vi "TCP Daemon.vi"(8 "UUID":string, 9 "Data Model":refnum<class "Device Data Model.lvclass">, 10 "transmission data unit":refnum<class "Transmission Data Unit.lvclass">, 11 "TCP slave in":refnum<class "TCP Slave.lvclass">) -> ()   [LabVIEW 2021, in "TCP Slave.lvclass"]
doc: "This daemon waits for new connections and launches connection handlers as needed. It also obtains a local reference to the quit notification, and waits for that to occur."
uses:
  TCP Slave.lvclass
  TCP Slave.lvclass/TCP Slave.ctl
  daemon status.ctl
  Network Slave.lvclass
  Listener State.ctl
  D:/my_projects/projects/Algorithms/Labview/21/Modbus_v21/Network Protocol/Network Slave/Network Slave.lvclass
  D:/my_projects/projects/Algorithms/Labview/21/Modbus_v21/Network Protocol/Network Protocol.lvclass
  D:/my_projects/projects/Algorithms/Labview/21/Modbus_v21/Network Protocol/Network Slave/TCP/TCP Slave.lvclass
  Data Model/Device Data Model.lvclass
  Transmission Data Unit/Transmission Data Unit.lvclass
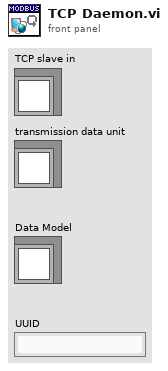
[diagram p1: front panel]
types:
  T1 = typedef "TCP Slave.lvclass/Listener State.ctl" = enum16{"Check Notifier", "Check for Available Connection Slot", "Wait on Connection", "Quit"}
  T2 = typedef "Network Slave.lvclass/daemon status.ctl" = enum16{"Not Started", "Running", "Error", "Stopped"}
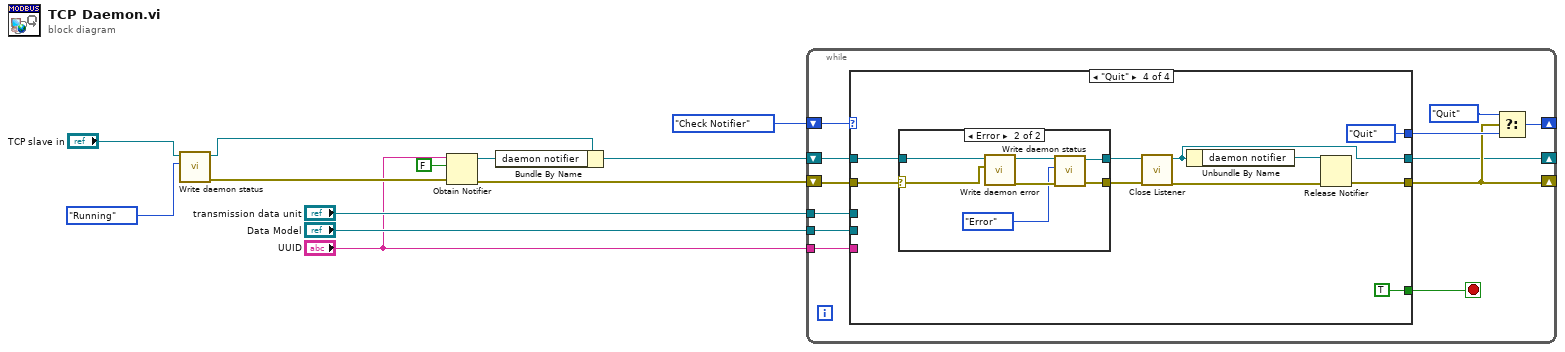
[diagram p0: block diagram]
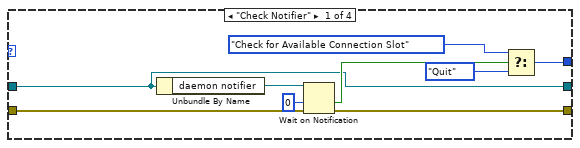
[diagram p2: hidden frame]
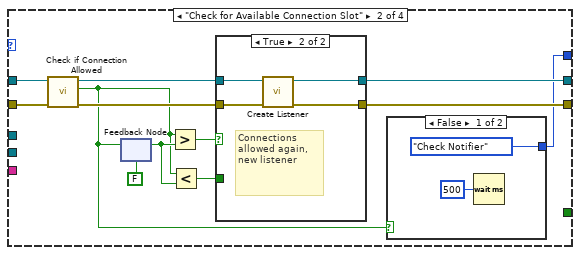
[diagram p3: hidden frame]
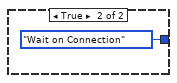
[diagram p4: hidden frame]
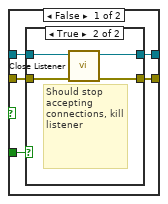
[diagram p5: hidden frame]
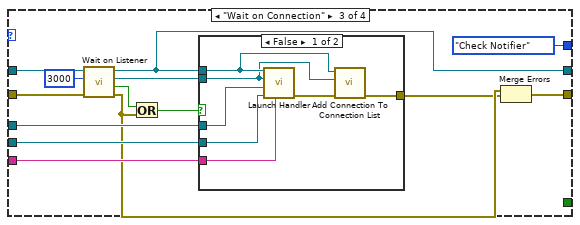
[diagram p7: hidden frame]
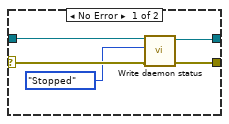
[diagram p9: hidden frame]
diagram:
  n1 = call "Write daemon status.vi"("daemon status"=daemon_status."Running", "Network Slave in"="TCP slave in") -> ("error out"=w6:errorcluster, "Network Slave out"=w7:refnum<class "TCP Slave.lvclass">)  [unwired: 8 in]
  n2 = Obtain Notifier(name (unnamed)="UUID", notification data type=FALSE, error in (no error)=w6) -> (notifier out=w10:refnum<notifier>, error out=w8:errorcluster)  [unwired: 1 in, 1 out]
  n3 = Bundle By Name(cluster=w7, "daemon notifier"=w10) -> (w9:refnum<class "TCP Slave.lvclass">)
  n4 = while {
    shift-right: [w22] -> _
    shift-left: Listener_State."Check Notifier" -> [w24]
    tunnel: "UUID" -> [w19]
    tunnel: "Data Model" -> [w18]
    tunnel: "transmission data unit" -> [w17]
    shift-right: [w16] -> _
    shift-left: w8 -> [w15]
    shift-right: [w13] -> _
    shift-left: w9 -> [w23]
    stop <- w14 stop-if-true
    n5 = case shown="\"Quit\"" w24 {
      tunnel: w23 -> [w25 w44 w76 w93]
      tunnel: [w32 w38 w66 w90] -> w16
      tunnel: [w27 w34 Listener_State."Check Notifier" Listener_State."Quit"] -> w20
      tunnel: w19 -> [_ _ w71 _]
      tunnel: w18 -> [_ _ w70 _]
      tunnel: w17 -> [_ _ w69 _]
      tunnel: w15 -> [w26 w45 w68 w94]
      tunnel: [_ _ _ TRUE] -> w14
      tunnel: [w25 w39 w67 w85] -> w13
      frame "Check Notifier" {
        n6 = Unbundle By Name(w25) -> ("daemon notifier"=w33:refnum<notifier>)
        n7 = Wait on Notification(notifier=w33, timeout in ms (-1)=0, error in (no error)=w26) -> (timed out?=w31:bool, error out=w32:errorcluster)  [unwired: 1 in, 2 out]
        n8 = Select(t=Listener_State."Check for Available Connection Slot", s=w31, f=Listener_State."Quit") -> (s? t:f=w27:T1)
      }
      frame "Check for Available Connection Slot" {
        n9 = call "Check if Connection Allowed.vi"("error in (no error)"=w45, "TCP Slave in"=w44) -> ("error out"=w41:errorcluster, "Connection Allowed"=w35:bool, "TCP Slave out"=w40:refnum<class "TCP Slave.lvclass">)  [unwired: 7 in]
        n10 = feedback-in #1(w35) -> ()
        n11 = feedback #1(FALSE) -> (w37:bool)
        n12 = Greater?(x=w35, y=w37) -> (0:w42:bool)
        n13 = Less?(x=w35, y=w37) -> (x < y?=w36:bool)
        n14 = case shown="True" w42 {
          tunnel: w41 -> [w51 w62]
          tunnel: w40 -> [w52 w63]
          tunnel: [w49 w61] -> w39
          tunnel: [w50 w60] -> w38
          tunnel: w36 -> [w53 _]
          frame False {
            n15 = case shown="True" w53 {
              tunnel: w52 -> [w55 w59]
              tunnel: w51 -> [w54 w58]
              tunnel: [w54 w57] -> w50
              tunnel: [w55 w56] -> w49
              frame False {
              }
              frame True {
                # "Should stop accepting connections, kill listener"
                n16 = call "Close Listener.vi"("error in"=w58, "TCP slave in"=w59) -> ("error out"=w57:errorcluster, "TCP slave out"=w56:refnum<class "TCP Slave.lvclass">)  [unwired: 8 in]
              }
            }
          }
          frame True {
            # "Connections allowed again, new listener"
            n17 = call "Create Listener.vi"("error in"=w62, "TCP slave in"=w63) -> ("error out"=w60:errorcluster, "TCP slave out"=w61:refnum<class "TCP Slave.lvclass">)  [unwired: 8 in]
          }
        }
        n18 = case shown="False" w35 {
          tunnel: [Listener_State."Check Notifier" Listener_State."Wait on Connection"] -> w34
          frame False {
            n19 = Wait (ms)(milliseconds to wait=u32 500) -> ()  [unwired: 1 out]
          }
          frame True {
          }
        }
      }
      frame "Wait on Connection" {
        n20 = call-dynamic "Wait on Listener.vi"("error in"=w68, "timeout ms (wait forever: -1)"=3000, "TCP slave in"=w76) -> ("error out"=w65:errorcluster, "Timed Out"=w74:bool, "connection reference"=w72:refnum<data-value>, "TCP slave out"=w67:refnum<class "TCP Slave.lvclass">)  [unwired: 5 in]
        n21 = Or(x=w74, y=w65) -> (x .or. y?=w73:bool)
        n22 = case shown="False" w73 {
          tunnel: w72 -> [w78 _]
          tunnel: w67 -> [w79 _]
          tunnel: w71 -> [w84 _]
          tunnel: w70 -> [w83 _]
          tunnel: w69 -> [w82 _]
          tunnel: [w81 _] -> w64
          frame False {
            n23 = call "Launch Handler.vi"("UUID"=w84, "Data Model"=w83, "transmission data unit"=w82, "connection reference"=w78, "TCP slave"=w79) -> ("error out"=w80:errorcluster)  [unwired: 6 in]
            n24 = call "Add Connection To Connection List.vi"("error in"=w80, "data value reference"=w78, "TCP Slave in"=w79) -> ("error out"=w81:errorcluster)  [unwired: 8 in]
          }
          frame True {
          }
        }
        n25 = Merge Errors(w65, w64) -> (w66:errorcluster)
      }
      frame "Quit" {
        n26 = case shown="Error" w94 {
          selector: w94 -> [w96 w101]
          tunnel: [w97 w103] -> w92
          tunnel: w93 -> [w99 w106]
          tunnel: [w98 w104] -> w91
          frame No Error {
            n27 = call "Write daemon status.vi"("error in (no error)"=w96, "daemon status"=daemon_status."Stopped", "Network Slave in"=w99) -> ("error out"=w97:errorcluster, "Network Slave out"=w98:refnum<class "TCP Slave.lvclass">)  [unwired: 7 in]
          }
          frame Error {
            n28 = call "Write daemon error.vi"("daemon error"=w101, "Network Slave in"=w106) -> ("error out"=w102:errorcluster, "Network Slave out"=w105:refnum<class "TCP Slave.lvclass">)  [unwired: 8 in]
            n29 = call "Write daemon status.vi"("error in (no error)"=w102, "daemon status"=daemon_status."Error", "Network Slave in"=w105) -> ("error out"=w103:errorcluster, "Network Slave out"=w104:refnum<class "TCP Slave.lvclass">)  [unwired: 7 in]
          }
        }
        n30 = call "Close Listener.vi"("error in"=w92, "TCP slave in"=w91) -> ("error out"=w86:errorcluster, "TCP slave out"=w85:refnum<class "TCP Slave.lvclass">)  [unwired: 8 in]
        n31 = Unbundle By Name(w85) -> ("daemon notifier"=w87:refnum<notifier>)
        n32 = Release Notifier(notifier=w87, error in (no error)=w86) -> (error out=w90:errorcluster)  [unwired: 1 in, 2 out]
      }
    }
    n33 = Select(t=Listener_State."Quit", s=w16, f=w20) -> (s? t:f=w22:T1)
  }
